vi "Disconnect.vi"(8 "error in (no error)":errorcluster, 11 "reference in":refnum<class "ZMQ_slave.lvclass">) -> (0 "error out":errorcluster, 3 "reference out":refnum<class "ZMQ_slave.lvclass">)   [LabVIEW 2019, in "CommandResponse communication.lvlib" / "ZMQ_slave.lvclass"]
doc: "Close all network streams to slave"
uses:
  ZMQ_slave.lvclass
  C:/Barkhausen mmWave radar/Development/LV/Barkhausen mmWave hardware control/Host/Intertarget communication/CR slave_class/CR slave.lvclass
  <vilib>/addons/zeromq/zmq_socket.lvclass
  <vilib>/addons/zeromq/zmq_context.lvclass
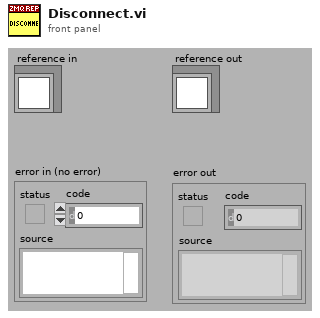
[diagram p1: front panel]
types:
  T1 = typedef "CommandResponse communication.lvlib/ZMQ_slave.lvclass/ObjectAttributes.ctl" = cluster{"ZMQ context":refnum<class "zmq_context.lvclass">, "ZMQ socket":refnum<class "zmq_socket.lvclass">, "endpoint":string}
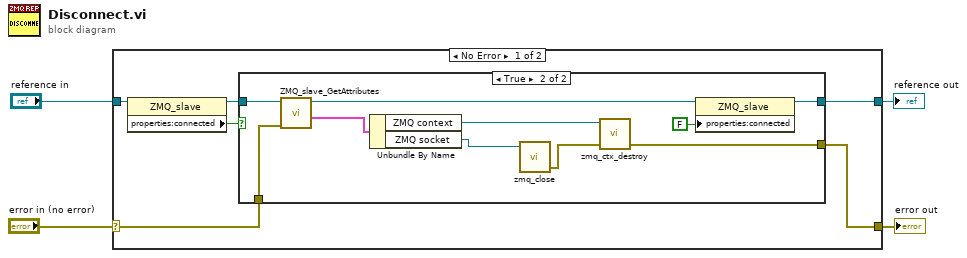
[diagram p0: block diagram]
diagram:
  n1 = case shown="No Error" "error in (no error)" {
    selector: "error in (no error)" -> [w10 w24]
    tunnel: [w7 w24] -> w3
    tunnel: [w9 w23] -> w1
    tunnel: "reference in" -> [w8 w23]
    frame No Error {
      n2 = property class="ZMQ_slave"(reference=w8) -> (reference out=w6:refnum<class "ZMQ_slave.lvclass">, "properties:connected"=w5:bool)  [unwired: 1 in, 1 out]
      n3 = case shown="True" w5 {
        tunnel: w10 -> [w11 w22]
        tunnel: [w12 w14] -> w9
        tunnel: [w11 w16] -> w7
        tunnel: w6 -> [w12 w15]
        frame False {
        }
        frame True {
          n4 = call "ZMQ_slave_GetAttributes.vi"("error in (no error)"=w22, "reference in"=w15) -> ("attributes"=w20:T1, "reference out"=w21:refnum<class "ZMQ_slave.lvclass">)  [unwired: 6 in, 2 out]
          n5 = Unbundle By Name(w20) -> ("ZMQ context"=w18:refnum<class "zmq_context.lvclass">, "ZMQ socket"=w19:refnum<class "zmq_socket.lvclass">)
          n6 = call <vilib>:"zmq_close.vi"("socket"=w19) -> ("error out"=w17:errorcluster)  [unwired: 4 in]
          n7 = call <vilib>:"zmq_ctx_destroy.vi"("error in"=w17, "context in"=w18) -> ("error out"=w16:errorcluster)  [unwired: 3 in]
          n8 = property class="ZMQ_slave"(reference=w21, "properties:connected"=FALSE) -> (reference out=w14:refnum<class "ZMQ_slave.lvclass">)  [unwired: 1 in, 1 out]
        }
      }
    }
    frame Error {
    }
  }
  "error out" <- w3
  "reference out" <- w1
